vi "K6485_init_filter.vi"(0 "Digital Filter Type (0: Repeating)":u16(ring) items=["Repeating", "Moving"], 1 "Digital Filter Noise Tolerance (0%)":dbl, 2 "Speedf (NPLC)[0.1-60]":string="1", 3 "Digital Filter Count (10)":i32=10, 4 "Enable Digital Filter (0: Disable)":u16(ring) items=["Disable", "Enable", "Advanced"], 5 "Address":string="14") -> ()   [LabVIEW 2021]
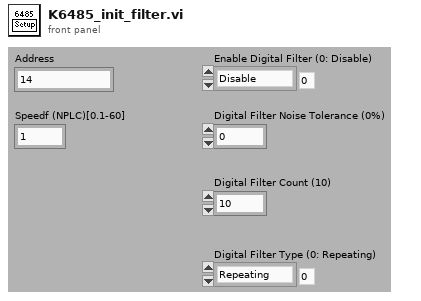
[diagram p1: front panel]
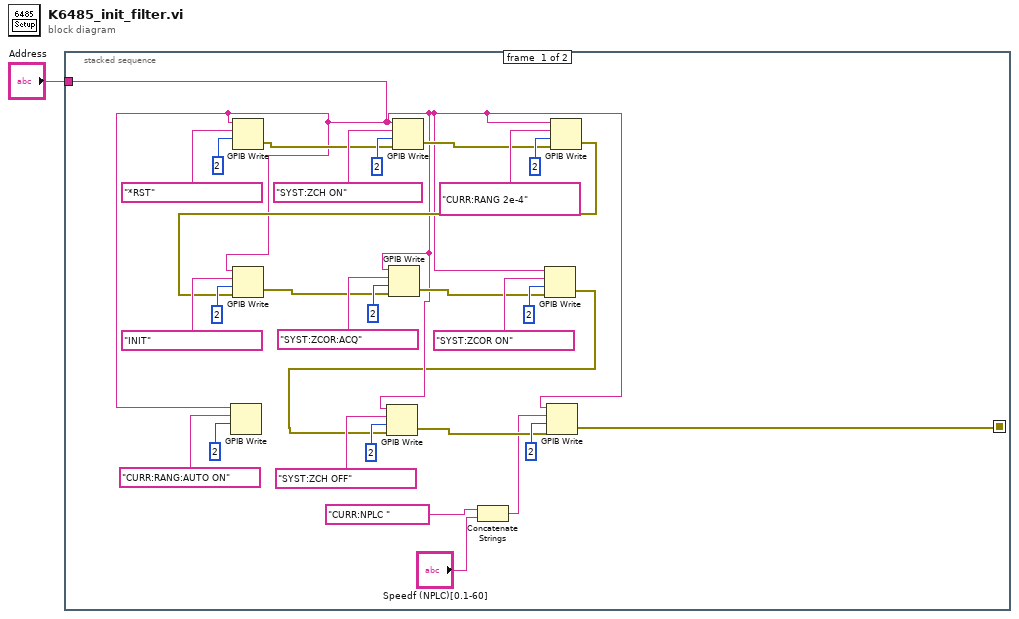
[diagram p0: block diagram]
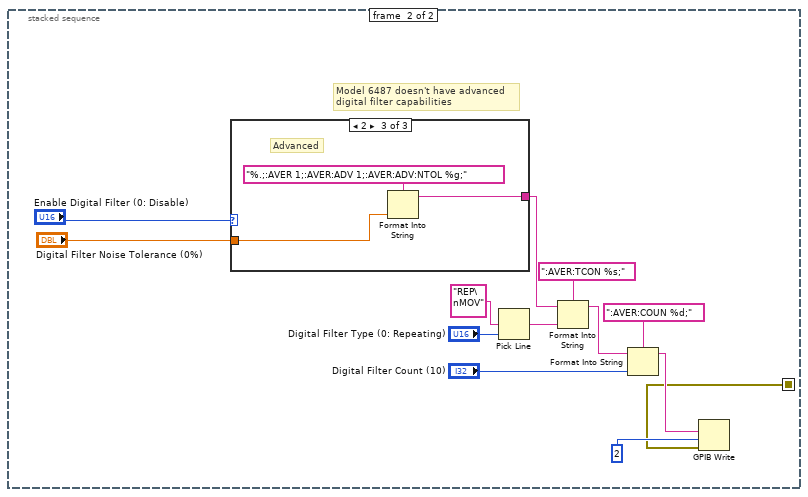
[diagram p2: hidden frame]
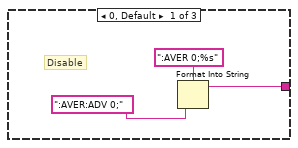
[diagram p3: hidden frame]
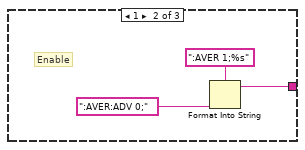
[diagram p4: hidden frame]
diagram:
  n1 = stacked-sequence {
    seq-local: [w3 _] -> [_ w31]
    tunnel: "Address" -> [w4 _]
    frame #0 {
      n2 = GPIB Write(0:w4, 1:"CURR:RANG:AUTO ON", 2:2) -> ()  [unwired: 2 in, 2 out]
      n3 = GPIB Write(0:w4, 1:"*RST", 2:2) -> (6:w26:errorcluster)  [unwired: 2 in, 1 out]
      n4 = GPIB Write(0:w4, 1:"SYST:ZCH ON", 2:2, 3:w26) -> (6:w23:errorcluster)  [unwired: 1 in, 1 out]
      n5 = Concatenate Strings("CURR:NPLC ", "Speedf (NPLC)[0.1-60]") -> (w5:string)
      n6 = GPIB Write(0:w4, 1:"CURR:RANG 2e-4", 2:2, 3:w23) -> (6:w17:errorcluster)  [unwired: 1 in, 1 out]
      n7 = GPIB Write(0:w4, 1:"INIT", 2:2, 3:w17) -> (6:w18:errorcluster)  [unwired: 1 in, 1 out]
      n8 = GPIB Write(0:w4, 1:"SYST:ZCOR:ACQ", 2:2, 3:w18) -> (6:w14:errorcluster)  [unwired: 1 in, 1 out]
      n9 = GPIB Write(0:w4, 1:"SYST:ZCOR ON", 2:2, 3:w14) -> (6:w2:errorcluster)  [unwired: 1 in, 1 out]
      n10 = GPIB Write(0:w4, 1:"SYST:ZCH OFF", 2:2, 3:w2) -> (6:w8:errorcluster)  [unwired: 1 in, 1 out]
      n11 = GPIB Write(0:w4, 1:w5, 2:2, 3:w8) -> (6:w3:errorcluster)  [unwired: 1 in, 1 out]
    }
    frame #1 {
      # "Model 6487 doesn't have advanced\ndigital filter capabilities"
      n12 = case shown="2" "Enable Digital Filter (0: Disable)" {
        tunnel: [w45 w48 w51] -> w41
        tunnel: "Digital Filter Noise Tolerance (0%)" -> [_ _ w50]
        frame 0, Default {
          # "Disable"
          n13 = Format Into String(format string=":AVER 0;%s", ":AVER:ADV 0;" ("t")) -> (resulting string=w45:string)  [unwired: 2 in, 1 out]
        }
        frame 1 {
          # "Enable"
          n14 = Format Into String(format string=":AVER 1;%s", ":AVER:ADV 0;" ("t")) -> (resulting string=w48:string)  [unwired: 2 in, 1 out]
        }
        frame 2 {
          # "Advanced"
          n15 = Format Into String(format string="%.;:AVER 1;:AVER:ADV 1;:AVER:ADV:NTOL %g;", w50) -> (resulting string=w51:string)  [unwired: 2 in, 1 out]
        }
      }
      n16 = Pick Line(multi-line string="REP\nMOV", line index="Digital Filter Type (0: Repeating)") -> (output string=w38:string)  [unwired: 1 in]
      n17 = Format Into String(format string=":AVER:TCON %s;", initial string=w41, w38) -> (resulting string=w36:string)  [unwired: 1 in, 1 out]
      n18 = Format Into String(format string=":AVER:COUN %d;", initial string=w36, "Digital Filter Count (10)") -> (resulting string=w32:string)  [unwired: 1 in, 1 out]
      n19 = GPIB Write(1:w32, 2:2, 3:w31) -> ()  [unwired: 2 in, 2 out]
    }
  }
